vi "test_MultipleSessionsReserved_InitializeSessions_SessionsAddedToConnectionMap.vi"(8 "error in":errorcluster) -> (0 "error out":errorcluster, 2 "result":string, 3 "pass":bool)   [LabVIEW 2020, in "MeasurementServerTests.lvlib"]
uses:
  MeasurementServerTests.lvlib
  Helpers/Fake Session Factory/Fake Session Factory.lvclass
  da6ffb6f-c1c9-4957-84dd-e9228483c454.vi
  a956f7ee-c7e9-4639-884c-f4265dae6ecf.vi
  Runtime/MeasurementLink Session Management V1/Session Reservation/Connection.ctl
  Runtime/MeasurementLink Session Management V1/Session Reservation/Session Reservation.lvclass
  Runtime/MeasurementLink Session Management V1/Session Reservation/Connection with Session.ctl
  9551059f-18af-4e23-b734-10739766adb6.vi
  Runtime/MeasurementLink Session Management V1/Session Reservation/Pin Type.ctl
  Runtime/MeasurementLink Session Management V1/Session Reservation/Initialize and Close Session Behavior.ctl
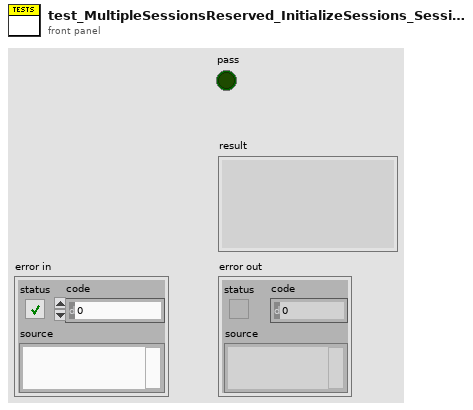
[diagram p1: front panel]
types:
  T1 = typedef "MeasurementLink Session Management V1.lvlib/Session Reservation.lvclass/Initialize and Close Session Behavior.ctl" = enum16{"Auto", "Initialize and Close", "Attach and Detach", "Initialize and Detach", "Attach and Close"}
  T2 = typedef "MeasurementLink Session Management V1.lvlib/Session Reservation.lvclass/Pin Type.ctl" = enum16{"DUT and System Pins", "System Pins"}
  T3 = typedef "MeasurementLink Session Management V1.lvlib/Session Reservation.lvclass/Connection with Session.ctl" = cluster{"connection":T4, "session":variant}
  T4 = typedef "MeasurementLink Session Management V1.lvlib/Session Reservation.lvclass/Connection.ctl" = cluster{"pin or relay name":string, "site":i32, "instrument type id":string, "channel":string}
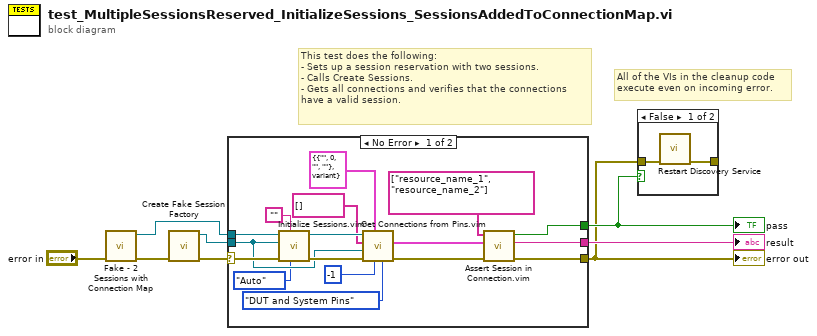
[diagram p0: block diagram]
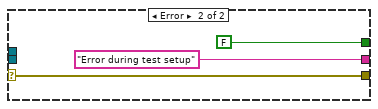
[diagram p2: hidden frame]
diagram:
  # "All of the VIs in the cleanup code\nexecute even on incoming error."
  # "This test does the following:\n- Sets up a session reservation with two sessions.\n- Calls Create Sessions.\n- Gets all connections and verifies that the connections\nhave a valid session."
  n1 = call "Fake - 2 Sessions with Connection Map.vi"("error in"="error in") -> ("error out"=w2:errorcluster, "session reservation out"=w1:refnum<class "Session Reservation.lvclass">)  [unwired: 9 in]
  n2 = call "Create Fake Session Factory.vi"("error in"=w2) -> ("error out"=w5:errorcluster, "fake session factory out"=w4:refnum<class "Fake Session Factory.lvclass">)  [unwired: 9 in]
  n3 = case shown="No Error" w5 {
    selector: w5 -> [w23 w25]
    tunnel: [w13 w25] -> w6
    tunnel: [w15 FALSE] -> w7
    tunnel: [w14 "Error during test setup" ("f")] -> w8
    tunnel: w4 -> [w18 _]
    tunnel: w1 -> [w24 _]
    frame No Error {
      n4 = call "Initialize Sessions.vim"("initialize and close session behavior"=Initialize_and_Close_Session_Behavior."Auto", "session type"="", "error in"=w23, "session factory"=w18, "session reservation in"=w24) -> ("error out"=w21:errorcluster, "session reservation out"=w20:refnum<class "Session Reservation.lvclass">)  [unwired: 3 in, 2 out]
      n5 = call "Get Connections from Pins.vim"("pin type"=Pin_Type."DUT and System Pins", "site"=-1, "connection type"=T3 {"connection"={"pin or relay name"="", "site"=0, "instrument type id"="", "channel"=""}, "session"=variant}, "error in"=w21, "session factory"=w18, "pin or relay names"=string[] [], "session reservation in"=w20) -> ("error out"=w13:errorcluster, "connections"=w12:T3[])  [unwired: 2 in, 1 out]
      n6 = call "Assert Session in Connection.vim"("actual connections"=w12, "expected session"=string[] ["resource_name_1", "resource_name_2"]) -> ("result"=w14:string, "pass"=w15:bool)  [unwired: 8 in]
    }
    frame Error {
    }
  }
  "error out" <- w6
  "pass" <- w7
  "result" <- w8
  n7 = case shown="False" w7 {
    tunnel: w6 -> [w29 _]
    tunnel: [w28 _] -> _
    frame False {
      n8 = call "Restart Discovery Service.vi"("error in"=w29) -> ("error out"=w28:errorcluster)  [unwired: 10 in]
    }
    frame True {
    }
  }
